vi "Pueba2 DAQ (2).vi"() -> ()   [LabVIEW 2011]
panel:
  in  "ON/OFF Temporal":bool
  in  "Brake Temporal":bool
  in  "Acelerar Temporal":bool
  in  "stop":bool
  out "Alarma de temp.":bool
  out "Meter":i32(knob) scale=0.0..5.0
  out "Cuarta":bool
  out "Tercera":bool
  out "Segunda":bool
  out "Primera":bool
  out "Brake":bool
  out "Acelerar":bool
  out "Velocidad":i32(knob) scale=0.0..220.0
  # "Se tiene que generar la temp del auto de acuerdo a la \nvelocidad:\n1-70 temp 1-2\n70-130 temp 1-4\n130- temp 1-5\nEsto es una entrada que se escribe en la temperatura\ny salida analogica que se ingresa del valor de la temp\nde la DAQ.\n\nEl acelerador cada vez que se pulsa el boton que sera\nuna entrada de la DAQ aumenta la velocidad en 10.\nSi se presiona el boton de brake se rebaja la velocidad en 5.\n\nDebera producirse 4 salidas digitales para representar\ncada uno de los cambios usando led\n1-30 primera\n31-50 segunda\n51-80 tercera\n80- cuarta\n\nLa alarma de la temperatura se enciende solo si esta sube\nde 3 enciende un led en la DAQ, ;a que es una salida\ndigital."
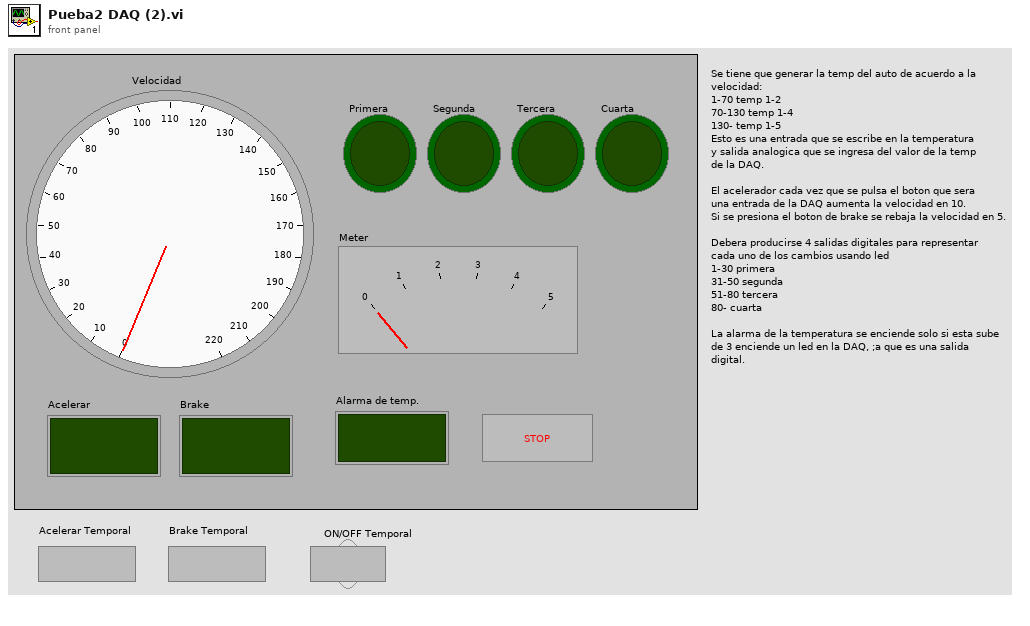
[diagram p1: front panel]
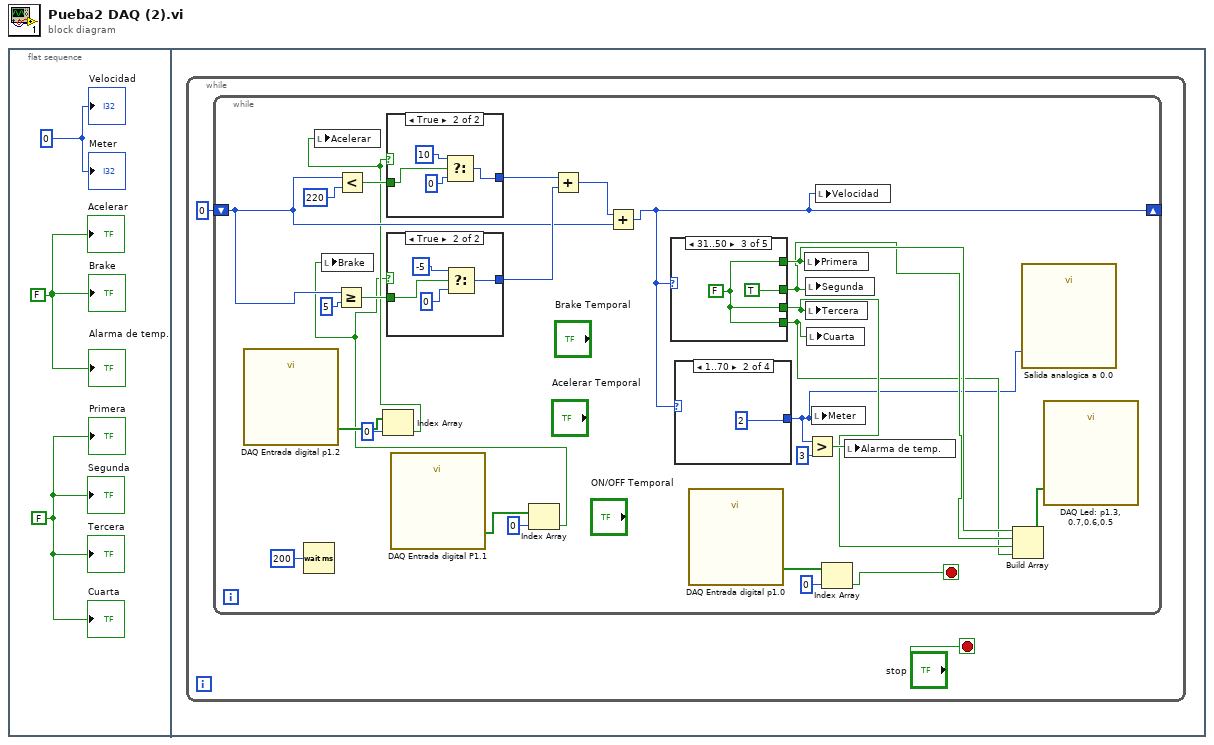
[diagram p0: block diagram]
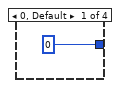
[diagram p2: hidden frame]
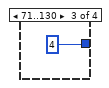
[diagram p3: hidden frame]
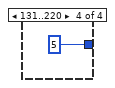
[diagram p4: hidden frame]
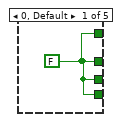
[diagram p5: hidden frame]
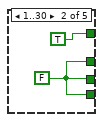
[diagram p6: hidden frame]
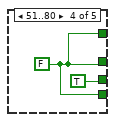
[diagram p7: hidden frame]
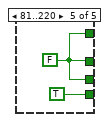
[diagram p8: hidden frame]
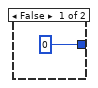
[diagram p9: hidden frame]
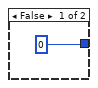
[diagram p10: hidden frame]
diagram:
  n1 = flat-sequence {
    frame #0 {
      w1 = FALSE
      w2 = FALSE
      w3 = 0
      "Velocidad" <- w3
      "Meter" <- w3
      "Acelerar" <- w2
      "Brake" <- w2
      "Alarma de temp." <- w2
      "Primera" <- w1
      "Segunda" <- w1
      "Tercera" <- w1
      "Cuarta" <- w1
    }
    frame #1 {
      n2 = while {
        stop <- "stop" stop-if-true
        n3 = while {
          shift-right: [w24] -> _
          shift-left: 0 -> [w25]
          stop <- w7 stop-if-true
          n4 = call "DAQ Entrada digital p1.2"() -> ("data"=w20:bool[])  [unwired: 17 in, 2 out]
          n5 = Wait (ms)(milliseconds to wait=u32 200) -> ()  [unwired: 1 out]
          n6 = Greater Or Equal?(x=w25, y=5) -> (x >= y?=w28:bool)
          n7 = Less?(x=w25, y=220) -> (x < y?=w31:bool)
          n8 = Index Array(array=w20, index=0) -> (element=w18:bool)
          n9 = local write "Acelerar"(w18) -> ()
          n10 = case shown="True" w18 {
            tunnel: w31 -> [_ w55]
            tunnel: [0 w52] -> w30
            frame False {
            }
            frame True {
              n11 = Select(t=10, s=w55, f=0) -> (s? t:f=w52:i32)
            }
          }
          n12 = call "DAQ Entrada digital P1.1"() -> ("data"=w17:bool[])  [unwired: 17 in, 2 out]
          n13 = Index Array(array=w17, index=0) -> (element=w15:bool)
          n14 = local write "Brake"(w15) -> ()
          n15 = case shown="True" w15 {
            tunnel: w28 -> [_ w48]
            tunnel: [0 w47] -> w27
            frame False {
            }
            frame True {
              n16 = Select(t=-5, s=w48, f=0) -> (s? t:f=w47:i32)
            }
          }
          n17 = Add(x=w30, y=w27) -> (x+y=w26:i32)
          n18 = Add(x=w26, y=w25) -> (x+y=w24:i32)
          n19 = case shown="31..50" w24 {
            tunnel: [w37 w38 TRUE w42 w45] -> w13
            tunnel: [w37 TRUE w40 w42 w45] -> w14
            tunnel: [w37 w38 w40 w42 TRUE] -> w11
            tunnel: [w37 w38 w40 TRUE w45] -> w12
            frame 0, Default {
              w37 = FALSE
            }
            frame 1..30 {
              w38 = FALSE
            }
            frame 31..50 {
              w40 = FALSE
            }
            frame 51..80 {
              w42 = FALSE
            }
            frame 81..220 {
              w45 = FALSE
            }
          }
          n20 = case shown="1..70" w24 {
            tunnel: [0 2 4 5] -> w6
            frame 0, Default {
            }
            frame 1..70 {
            }
            frame 71..130 {
            }
            frame 131..220 {
            }
          }
          n21 = call "DAQ Entrada digital p1.0"() -> ("data"=w9:bool[])  [unwired: 17 in, 2 out]
          n22 = local write "Primera"(w14) -> ()
          n23 = local write "Segunda"(w13) -> ()
          n24 = local write "Tercera"(w12) -> ()
          n25 = local write "Cuarta"(w11) -> ()
          n26 = Greater?(x=w6, y=3) -> (0:w21:bool)
          n27 = local write "Meter"(w6) -> ()
          n28 = local write "Velocidad"(w24) -> ()
          n29 = Index Array(array=w9, index=0) -> (element=w7:bool)
          n30 = local write "Alarma de temp."(w21) -> ()
          n31 = Build Array(w14, w13, w12, w11) -> (w10:bool[])
          n32 = call "Salida analogica a 0.0"("data"=w6) -> ()  [unwired: 17 in, 2 out]
          n33 = call "DAQ Led: p1.3, 0.7,0.6,0.5"("data"=w10) -> ()  [unwired: 17 in, 2 out]
        }
      }
    }
  }
